vi "cluster unbundlele feb 11.vi"() -> ()   [LabVIEW 2015]
panel:
  out "Array 4":cluster{"Numeric":dbl, "Numeric 2":dbl}[](array[cluster])
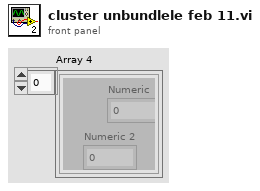
[diagram p1: front panel]
types:
  T1 = cluster{"[0]":void, "[1]":void, "[2]":void, "[3]":void, "[4]":void, "[5]":void, "[6]":void, "[7]":void, "[8]":void}
  T2 = cluster{cluster{"subarray[0]":dbl, "subarray[1]":dbl}, cluster{"subarray[2]":dbl, "subarray[3]":dbl}, cluster{"subarray[4]":dbl, "subarray[5]":dbl}}
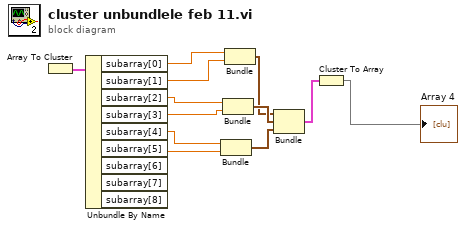
[diagram p0: block diagram]
diagram:
  n1 = Array To Cluster() -> (cluster=w2:T1)  [unwired: 1 in]
  n2 = Unbundle By Name(w2) -> ("subarray[0]"=w4:dbl, "subarray[1]"=w3:dbl, "subarray[2]"=w5:dbl, "subarray[3]"=w6:dbl, "subarray[4]"=w7:dbl, "subarray[5]"=w8:dbl)  [unwired: 3 out]
  n3 = Bundle("subarray[4]"=w7, "subarray[5]"=w8) -> (w11:cluster{"subarray[4]":dbl, "subarray[5]":dbl})  [unwired: 1 in]
  n4 = Bundle("subarray[2]"=w5, "subarray[3]"=w6) -> (w10:cluster{"subarray[2]":dbl, "subarray[3]":dbl})  [unwired: 1 in]
  n5 = Bundle("subarray[0]"=w4, "subarray[1]"=w3) -> (w9:cluster{"subarray[0]":dbl, "subarray[1]":dbl})  [unwired: 1 in]
  n6 = Bundle(w9, w10, w11) -> (w12:T2)  [unwired: 1 in]
  n7 = Cluster To Array(cluster=w12) -> (array=→"Array 4":cluster{"subarray[4]":dbl, "subarray[5]":dbl}[])
